vi "Format With Base System Image.vi"(4 "Base System Image":T1 {"component type" items=["standard", "hidden", "system", "unknown", "startup", "image", "essential"]}, 6 "Timeout (300,000 ms)":u32=300000, 7 "Restart Automatically (T)":bool=TRUE, 8 "error in (no error)":errorcluster, 9 "Network Settings (reset all adapters)":T3 items=["reset all network adapters", "preserve primary, reset others", "preserve all network adapters"], 10 "File System":T4 items=["Default"=0, "FAT"=1, "Reliance"=2, "UBIFS"=16384, "Ext4"=32768], 11 "Session in":refnum<k21>) -> (0 "error out":errorcluster, 3 "Session out":refnum<k21>)   [LabVIEW 2020, in "nisyscfg.lvlib"]
doc: "Erases all data from the primary hard drive of a system. The operation will fail if you choose not to restart the target automatically and the target's boot flow requires it to be in safe mode or restart after the operation. Refer to the the definition of safe mode to understand the differences between safe mode for different target boot flows."
uses:
  <vilib>/nisyscfg/nisyscfg.lvlib
  <vilib>/nisyscfg/File System.ctl
  <vilib>/nisyscfg/Network Settings Format.ctl
  <vilib>/nisyscfg/Software 1.2.ctl
  <vilib>/nisyscfg/Component Type.ctl
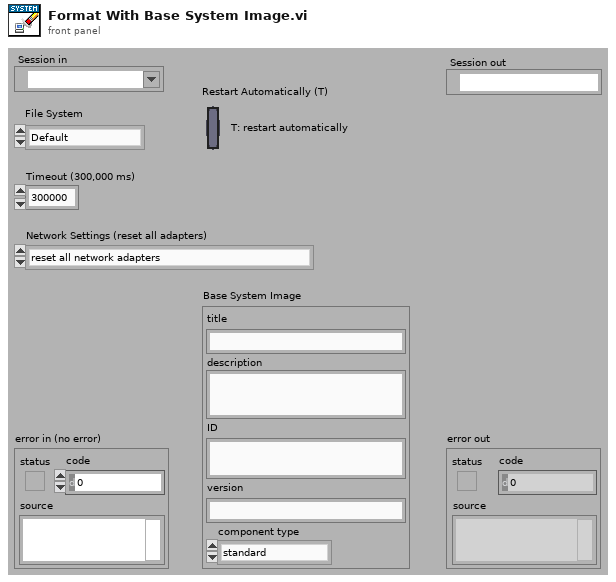
[diagram p1: front panel]
types:
  T1 = typedef "nisyscfg.lvlib/Software 1.2.ctl" = cluster{"title":string, "description":string, "ID":string, "version":string, "component type":T2}
  T2 = typedef "nisyscfg.lvlib/Component Type.ctl" = u32
  T3 = typedef "nisyscfg.lvlib/Network Settings Format.ctl" = u32
  T4 = typedef "nisyscfg.lvlib/File System.ctl" = i32
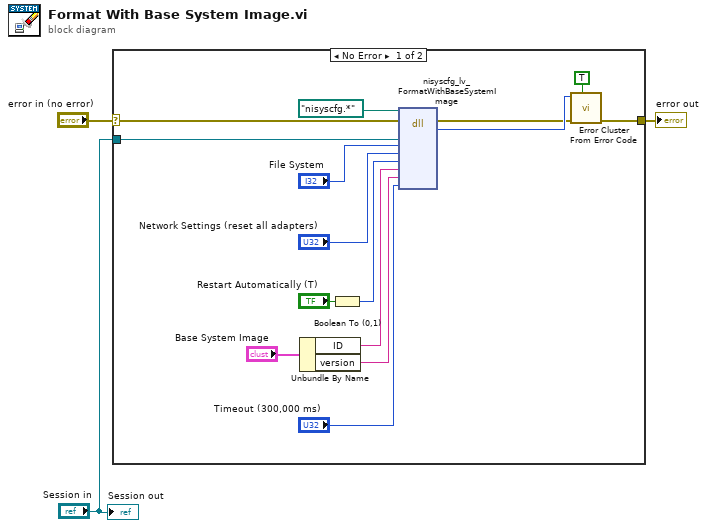
[diagram p0: block diagram]
diagram:
  n1 = case shown="No Error" "error in (no error)" {
    selector: "error in (no error)" -> [w12 w19]
    tunnel: "Session in" -> [w11 _]
    tunnel: [w10 w19] -> w3
    frame No Error {
      n2 = Unbundle By Name("Base System Image") -> ("ID"=w5:string, "version"=w4:string)
      n3 = Boolean To (0,1)(Boolean="Restart Automatically (T)") -> (0, 1=w9:i16)
      n4 = dll-call lib="nisyscfg.*" fn="nisyscfg_lv_FormatWithBaseSystemImage" label="FormatWithBaseSystemImage"(path in=path "nisyscfg.*", error in=w12, "system"=w11, "fileSystem"="File System", "networkSettings"="Network Settings (reset all adapters)", "autoRestart"=w9, "systemSetID"=w5, "systemSetVersion"=w4, "timeout"="Timeout (300,000 ms)") -> (error out=w17:errorcluster, "result"=w18:i32)  [unwired: 8 in, 1 out]
      n5 = call <vilib>:"Error Cluster From Error Code.vi"("show call chain? (False)"=TRUE, "error in (no error)"=w17, "error code (0)"=w18) -> ("error out"=w10:errorcluster)  [unwired: 6 in]
    }
    frame Error {
    }
  }
  "error out" <- w3
  "Session out" <- "Session in"
